vi "test.vi"() -> ()   [LabVIEW 2019]
uses:
  lvsrc/ProjectItem/ProjectItem.lvclass
panel:
  in  "Pattern":string="Template"
  in  "New Name":string="NewName"
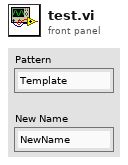
[diagram p1: front panel]
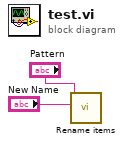
[diagram p0: block diagram]
diagram:
  n1 = call "Rename items.vi"("New Name"="New Name", "Pattern"="Pattern") -> ()  [unwired: 10 in]
